vi "checkPython.vi"() -> ()   [LabVIEW 2015]
panel:
  out "status_bar":string="Finalize\nCosmedAPTools installation....."
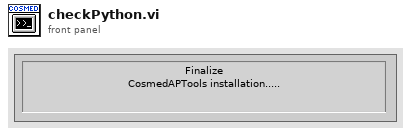
[diagram p1: front panel]
types:
  T1 = enum32{"invalid app kind", "Development System", "Run Time System", "Student Edition", "Embedded LabVIEW", "Evaluation", "Custom"}
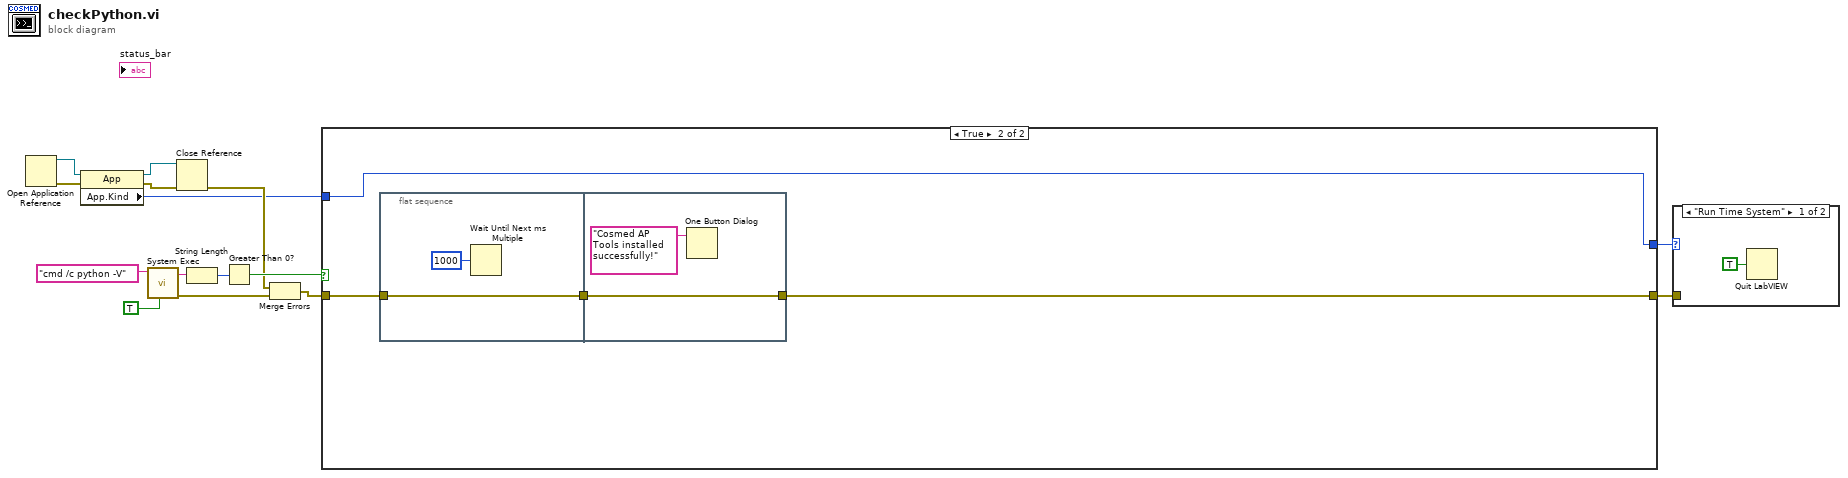
[diagram p0: block diagram]
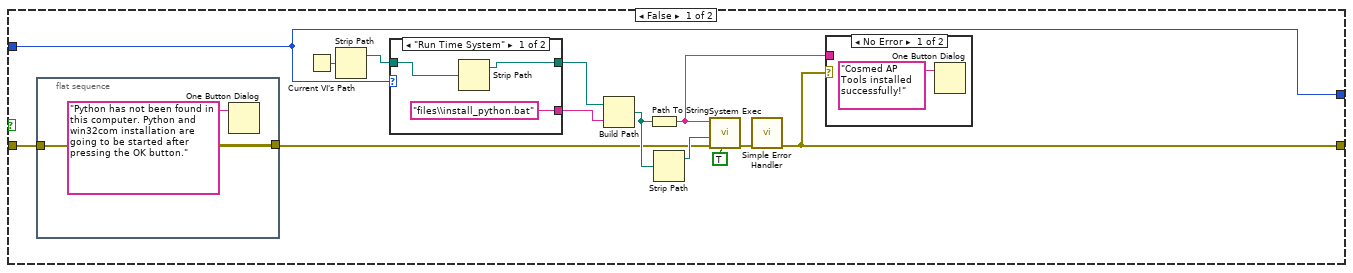
[diagram p3: hidden frame]
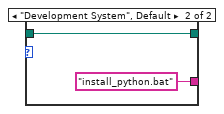
[diagram p4: hidden frame]
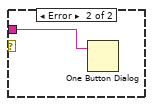
[diagram p5: hidden frame]
diagram:
  n1 = Open Application Reference() -> (0:w10:errorcluster, 3:w9:refnum<vi>)  [unwired: 4 in]
  n2 = property class="App"(reference=w9, error in=w10) -> (reference out=w7:refnum<vi>, error out=w8:errorcluster, "App.Kind"=w3:T1)
  n3 = call <vilib>:"System Exec.vi"("run minimized? (F)"=TRUE, "command line"="cmd /c python -V") -> ("error out"=w6:errorcluster, "standard output"=w14:string)  [unwired: 4 in, 4 out]
  n4 = Close Reference(reference=w7, error in (no error)=w8) -> (error out=w4:errorcluster)
  n5 = String Length(string=w14) -> (length=w13:i32)
  n6 = Greater Than 0?(x=w13) -> (x > 0?=w11:bool)
  n7 = Merge Errors(w4, w6) -> (w5:errorcluster)
  n8 = case shown="True" w11 {
    tunnel: w5 -> [w28 w41]
    tunnel: w3 -> [w16 w38]
    tunnel: [w17 w39] -> w2
    tunnel: [w16 w38] -> w1
    frame False {
      n9 = flat-sequence {
        tunnel: w28 -> [w36]
        tunnel: [w36] -> w18
        frame #0 {
          n10 = One Button Dialog(message="Python has not been found in this computer. Python and win32com installation are going to be started after pressing the OK button.") -> ()  [unwired: 1 in, 1 out]
        }
      }
      n11 = Current VI's Path() -> (path=w27:path)
      n12 = Strip Path(path=w27) -> (stripped path=w20:path)  [unwired: 1 out]
      n13 = case shown="\"Run Time System\"" w16 {
        tunnel: ["files\\install_python.bat" ("command line") "install_python.bat" ("command line")] -> w23
        tunnel: w20 -> [w30 w32]
        tunnel: [w29 w32] -> w19
        frame "Run Time System" {
          n14 = Strip Path(path=w30) -> (stripped path=w29:path)  [unwired: 1 out]
        }
        frame "Development System", Default {
        }
      }
      n15 = Build Path(base path=w19, name or relative path=w23) -> (appended path=w22:path)
      n16 = Path To String(path=w22) -> (string=w24:string)
      n17 = Strip Path(path=w22) -> (stripped path=w21:path)  [unwired: 1 out]
      n18 = call <vilib>:"System Exec.vi"("run minimized? (F)"=TRUE, "error in (no error)"=w18, "working directory"=w21, "command line"=w24) -> ("error out"=w26:errorcluster)  [unwired: 2 in, 5 out]
      n19 = call <vilib>:"Simple Error Handler.vi"("error in (no error)"=w26) -> ("error out"=w17:errorcluster)  [unwired: 4 in, 4 out]
      n20 = case shown="No Error" w17 {
        tunnel: w24 -> [_ w35]
        frame No Error {
          n21 = One Button Dialog(message="Cosmed AP Tools installed successfully!") -> ()  [unwired: 1 in, 1 out]
        }
        frame Error {
          n22 = One Button Dialog(message=w35) -> ()  [unwired: 1 in, 1 out]
        }
      }
    }
    frame True {
      n23 = flat-sequence {
        tunnel: w41 -> [w42]
        tunnel: [w42] -> w40
        tunnel: [w44] -> w39
        tunnel: w40 -> [w44]
        frame #0 {
          n24 = Wait Until Next ms Multiple(millisecond multiple=u32 1000) -> ()  [unwired: 1 out]
        }
        frame #1 {
          n25 = One Button Dialog(message="Cosmed AP Tools installed successfully!") -> ()  [unwired: 1 in, 1 out]
        }
      }
    }
  }
  n26 = case shown="\"Run Time System\"" w1 {
    tunnel: w2 -> [_ _]
    frame "Run Time System" {
      n27 = Quit LabVIEW(quit? (T)=TRUE) -> ()
    }
    frame "Development System", Default {
    }
  }
